vi "getTicksSinceOrigin.vi"(8 "error in (no error)":errorcluster, 11 "IDevice in":refnum<class "IDevice.lvclass">) -> (0 "error out":errorcluster, 2 "Ticks Since Origin out":u64, 3 "IDevice out":refnum<class "IDevice.lvclass">)   [LabVIEW 2022 SP3, in "openDAQ.lvlib" / "IBaseObject.lvlib" / "IPropertyObject.lvlib" / "IComponent.lvlib" / "IFolder.lvlib" / "IDevice.lvlib" / "IDevice.lvclass"]
uses:
  <instrlib>/openDAQ/Public/Classes/IDevice/IDevice.lvclass
  <instrlib>/openDAQ/Public/Classes/IDevice/IDevice.lvclass/IDevice.ctl
  <instrlib>/openDAQ/Binaries/Windows/x86/copendaq32.dll
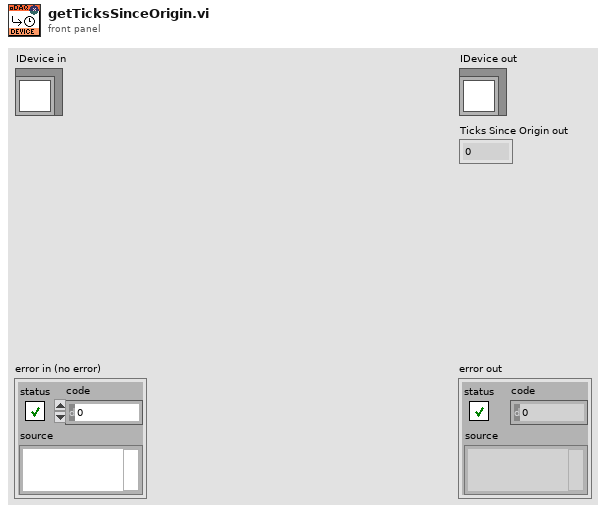
[diagram p1: front panel]
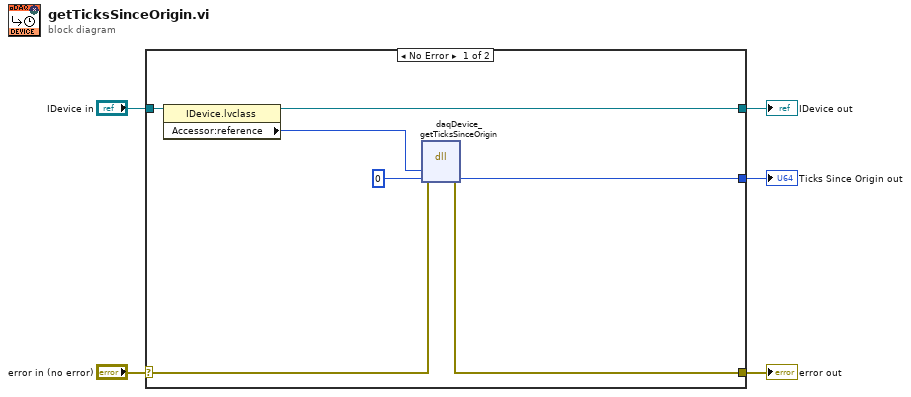
[diagram p0: block diagram]
diagram:
  n1 = case shown="No Error" "error in (no error)" {
    selector: "error in (no error)" -> [w10 w14]
    tunnel: [w9 w14] -> w4
    tunnel: [w8 w13] -> w2
    tunnel: "IDevice in" -> [w12 w13]
    tunnel: [w7 _] -> w1
    frame No Error {
      n2 = property class="IDevice.lvclass"(reference=w12) -> (reference out=w8:refnum<class "IDevice.lvclass">, "Accessor:reference"=w11:i64)  [unwired: 1 in, 1 out]
      n3 = dll-call lib="C:/Program Files (x86)/National Instruments/LabVIEW 2022/instr.lib/openDAQ/Binaries/Windows/x86/copendaq*.*" fn="daqDevice_getTicksSinceOrigin"(error in=w10, "device"=w11, "ticks"=u64 0) -> (error out=w9:errorcluster, "ticks"=w7:u64)  [unwired: 4 in, 1 out]
    }
    frame Error {
    }
  }
  "error out" <- w4
  "IDevice out" <- w2
  "Ticks Since Origin out" <- w1
